vi "Module Cleanup.vi"(8 "error in (no error)":errorcluster, 11 "Config Alert Module in":refnum<class "Config Monitor Module.lvclass">) -> (0 "error out":errorcluster, 3 "Config Alert Module out":refnum<class "Config Monitor Module.lvclass">)   [LabVIEW 2020, in "Volatus.lvlib" / "Config Monitor Module.lvclass"]
uses:
  Config Monitor Module.lvclass
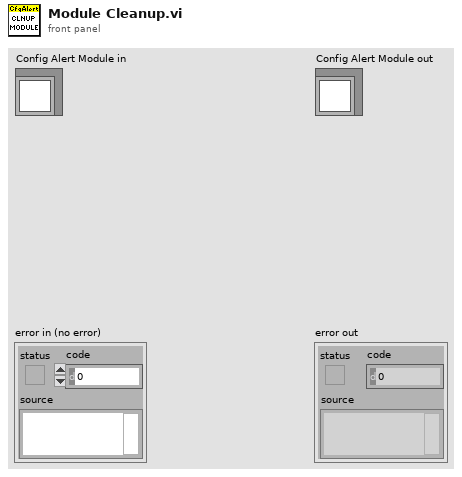
[diagram p1: front panel]
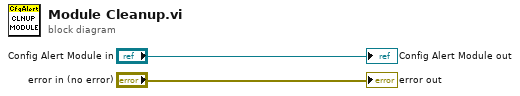
[diagram p0: block diagram]
diagram:
  "error out" <- "error in (no error)"
  "Config Alert Module out" <- "Config Alert Module in"
